vi "PhotonUtils_GetTargetById.vi"(10 "PhotonPipelineResult":T6 {"Targets"."CameraToTarget"."ROTATION"."SIN" format="%13.4f"; "Targets"."CameraToTarget"."ROTATION"."COS" format="%13.4f"; "Targets"."CameraToTarget"."ROTATION"."VALUE" format="%13.4f"; "Targets"."CameraToTarget"."TRANSLATION"."Y" format="%14.3f"; "Targets"."CameraToTarget"."TRANSLATION"."X" format="%14.3f"}, 11 "FiducialId":i32) -> (2 "Found Target?":bool, 3 "PhotonTrackedTarget":T1={"Yaw"=0.0, "Pitch"=0.0, "Area"=0.0, "Skew"=0.0, "TargetCorners"=[], "CameraToTarget"={"TRANSLATION"={"X"=0.0, "Y"=0.0}, "ROTATION"={"VALUE"=0.0, "COS"=1.0, "SIN"=0.0}, "xF"=FALSE}, "FiducialId"=0} {"CameraToTarget"."ROTATION"."SIN" format="%13.4f"; "CameraToTarget"."ROTATION"."COS" format="%13.4f"; "CameraToTarget"."ROTATION"."VALUE" format="%13.4f"; "CameraToTarget"."TRANSLATION"."Y" format="%14.3f"; "CameraToTarget"."TRANSLATION"."X" format="%14.3f"})   [LabVIEW 2020, in "PhotonVisionLib.lvlib"]
uses:
  PhotonVisionLib.lvlib
  TypeDef/PhotonPipelineResultType.ctl
  TypeDef/PhotonTrackedTargetType.ctl
  TypeDef/TargetCornerType.ctl
  <vilib>/Rock Robotics/WPI/ThirdParty/JAS_Junk/TrajLib/TypeDef/TRANSFORM2D.ctl
  <vilib>/Rock Robotics/WPI/ThirdParty/JAS_Junk/TrajLib/TypeDef/TRANSLATION2D.ctl
  <vilib>/Rock Robotics/WPI/ThirdParty/JAS_Junk/TrajLib/TypeDef/ROTATION2D.ctl
  <vilib>/Rock Robotics/WPI/ThirdParty/JAS_Junk/TrajLib/Trajectory_Library.lvlib
panel:
  in  "target index":i32
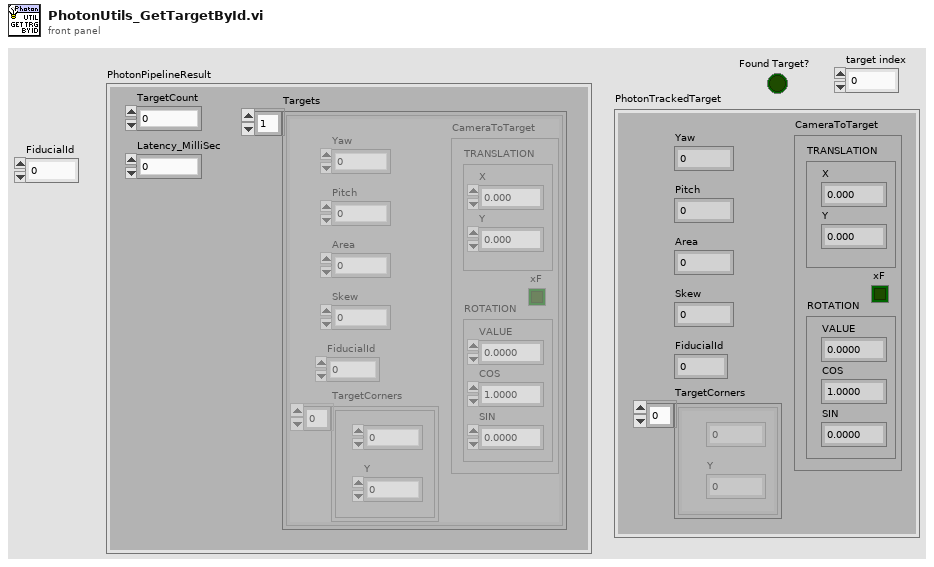
[diagram p1: front panel]
types:
  T1 = typedef "PhotonVisionLib.lvlib/PhotonTrackedTargetType.ctl" = cluster{"Yaw":dbl, "Pitch":dbl, "Area":dbl, "Skew":dbl, "TargetCorners":T2[], "CameraToTarget":T3, "FiducialId":i32}
  T2 = typedef "PhotonVisionLib.lvlib/TargetCornerType.ctl" = cluster{"X":dbl, "Y":dbl}
  T3 = typedef "Trajectory_Library.lvlib/TRANSFORM2D.ctl" = cluster{"TRANSLATION":T4, "ROTATION":T5, "xF":bool}
  T4 = typedef "Trajectory_Library.lvlib/TRANSLATION2D.ctl" = cluster{"X":dbl, "Y":dbl}
  T5 = typedef "Trajectory_Library.lvlib/ROTATION2D.ctl" = cluster{"VALUE":dbl, "COS":dbl, "SIN":dbl}
  T6 = typedef "PhotonVisionLib.lvlib/PhotonPipelineResultType.ctl" = cluster{"TargetCount":i32, "Latency_MilliSec":dbl, "Targets":T1[]}
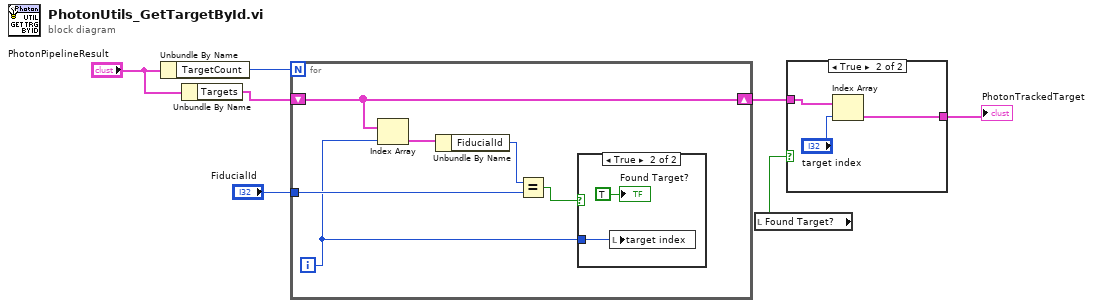
[diagram p0: block diagram]
diagram:
  n1 = Unbundle By Name("PhotonPipelineResult") -> ("TargetCount"=w7:i32)
  n2 = Unbundle By Name("PhotonPipelineResult") -> ("Targets"=w4:T1[])
  n3 = for {
    N: w7 -> [_]
    tunnel: "FiducialId" -> [w13]
    shift-right: [w12] -> w2
    shift-left: w4 -> [w12]
    i -> [w8]
    n4 = Index Array(array=w12, index=w8) -> (element=w11:T1)
    n5 = Unbundle By Name(w11) -> ("FiducialId"=w10:i32)
    n6 = Equal?(x=w10, y=w13) -> (x = y?=w9:bool)
    n7 = case shown="True" w9 {
      tunnel: w8 -> [_ w14]
      frame False {
      }
      frame True {
        n8 = local write "target index"(w14) -> ()
        "Found Target?" <- TRUE ("Found Target?")
      }
    }
  }
  n9 = local read "Found Target?"() -> (w3:bool)
  n10 = case shown="True" w3 {
    tunnel: w2 -> [_ w18]
    tunnel: [_ w16] -> w1
    frame False {
    }
    frame True {
      n11 = Index Array(array=w18, index="target index") -> (element=w16:T1)
    }
  }
  "PhotonTrackedTarget" <- w1
